vi "rekawica.vi"(7 "VISA resource name":refnum<visa-resource-name>, 8 "StartReading":bool) -> ()   [LabVIEW 2017]
uses:
  <vilib>/Instr/_visa.llb/VISA Configure Serial Port (Instr).vi
panel:
  out "Y":i32
  out "X":i32
  out "palec5":i32
  out "palec4":i32
  out "pale3":i32
  out "palec2":i32
  out "palec1":i32
  out "readBuffor":string
  in  "STOP":bool
  # "Dane przesyłane do łazika"
  # "Dane odbierane z rekawicy"
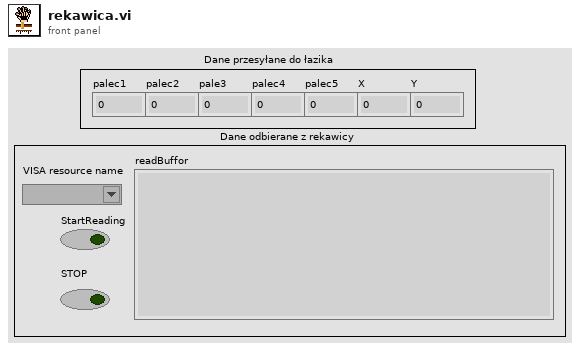
[diagram p1: front panel]
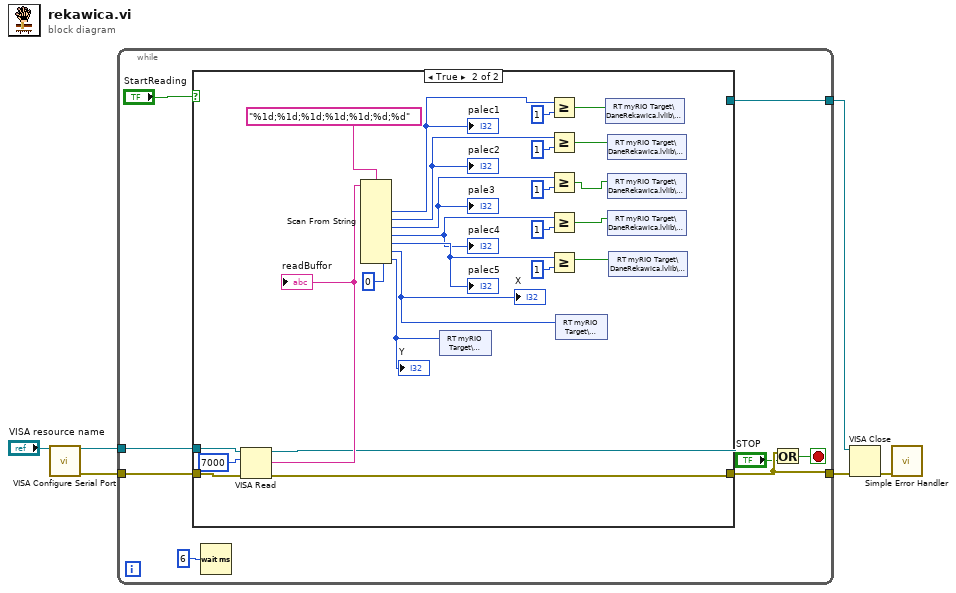
[diagram p0: block diagram]
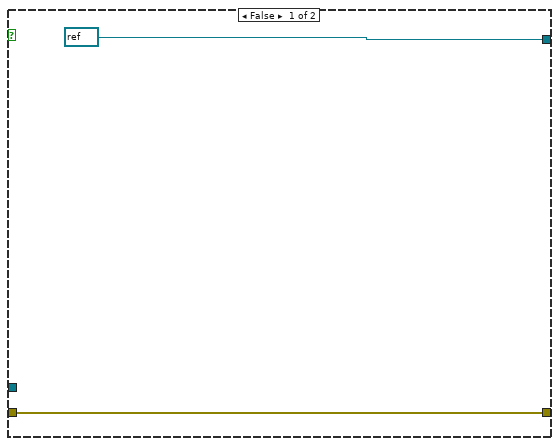
[diagram p2: hidden frame]
diagram:
  n1 = call-poly "VISA Configure Serial Port"("VISA resource name"="VISA resource name") -> ("VISA resource name out"=w4:refnum<visa-resource-name>, "error out"=w5:errorcluster)  [unwired: 13 in]
  n2 = while {
    tunnel: w5 -> [w13]
    tunnel: w4 -> [w12]
    tunnel: [w10] -> w3
    tunnel: [w7] -> w2
    stop <- w11 stop-if-true
    n3 = case shown="True" "StartReading" {
      tunnel: w13 -> [w16 w41]
      tunnel: w12 -> [_ w40]
      tunnel: [w16 w38] -> w10
      tunnel: [refnum<visa-resource-name> refnum ("VISA resource name out") w34] -> w7
      frame False {
      }
      frame True {
        w35 = 0
        n4 = VISA Read(VISA resource name=w40, byte count=u32 7000 ("Read Count"), error in (no error)=w41) -> (VISA resource name out=w34:refnum<visa-resource-name>, read buffer=w37:string, error out=w38:errorcluster)  [unwired: 1 out]
        "readBuffor" <- w37
        n5 = Scan From String(format string="%1d;%1d;%1d;%1d;%1d;%d;%d", input string=w37, default 1=w35, default 2=w35, default 3=w35, default 4=w35, default 5=w35, default 6=w35, default 7=w35) -> (output 1=w33:i32, output 2=w24:i32, output 3=w25:i32, output 4=w26:i32, output 5=w27:i32, output 6=w21:i32, output 7=w22:i32)  [unwired: 2 in, 3 out]
        "palec2" <- w24
        "pale3" <- w25
        "palec4" <- w26
        "palec5" <- w27
        "X" <- w21
        "Y" <- w22
        "palec1" <- w33
        n6 = shared-variable "RT myRIO Target\\DaneRekawica.lvlib\\Y"(w22) -> ()  [unwired: 1 in, 1 out]
        n7 = Greater Or Equal?(x=w33, y=1) -> (x >= y?=w23:bool)
        n8 = Greater Or Equal?(x=w24, y=1) -> (x >= y?=w17:bool)
        n9 = Greater Or Equal?(x=w25, y=1) -> (x >= y?=w18:bool)
        n10 = Greater Or Equal?(x=w26, y=1) -> (x >= y?=w19:bool)
        n11 = Greater Or Equal?(x=w27, y=1) -> (x >= y?=w20:bool)
        n12 = shared-variable "RT myRIO Target\\DaneRekawica.lvlib\\X"(w21) -> ()  [unwired: 1 in, 1 out]
        n13 = shared-variable "RT myRIO Target\\DaneRekawica.lvlib\\Palec1"(w23) -> ()  [unwired: 1 in, 1 out]
        n14 = shared-variable "RT myRIO Target\\DaneRekawica.lvlib\\Palec2"(w17) -> ()  [unwired: 1 in, 1 out]
        n15 = shared-variable "RT myRIO Target\\DaneRekawica.lvlib\\Palec3"(w18) -> ()  [unwired: 1 in, 1 out]
        n16 = shared-variable "RT myRIO Target\\DaneRekawica.lvlib\\Palec4"(w19) -> ()  [unwired: 1 in, 1 out]
        n17 = shared-variable "RT myRIO Target\\DaneRekawica.lvlib\\Palec5"(w20) -> ()  [unwired: 1 in, 1 out]
      }
    }
    n18 = Wait (ms)(milliseconds to wait=u32 6) -> ()  [unwired: 1 out]
    n19 = Or(x=w10, y="STOP") -> (x .or. y?=w11:bool)
  }
  n20 = VISA Close(VISA resource name=w2, error in (no error)=w3) -> (error out=w1:errorcluster)
  n21 = call <vilib>:"Simple Error Handler.vi"("error in (no error)"=w1) -> ()  [unwired: 4 in, 5 out]
